vi "_23_Sample_qsns_10[3].vi"() -> ()   [LabVIEW 2020]
panel:
  out "s? t:f":dbl
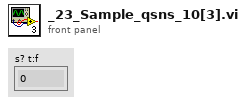
[diagram p1: front panel]
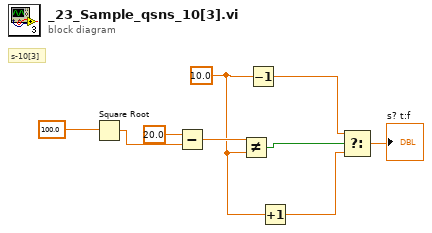
[diagram p0: block diagram]
diagram:
  w5 = 10.0 ("x")
  # "s-10[3]"
  n1 = Square Root(x=100.0) -> (sqrt(x)=w8:dbl)
  n2 = Subtract(x=20.0, y=w8) -> (x-y=w6:dbl)
  n3 = Not Equal?(x=w6, y=w5) -> (x != y?=w4:bool)
  n4 = Decrement(x=w5) -> (x-1=w3:dbl)
  n5 = Increment(x=w5) -> (x+1=w2:dbl)
  n6 = Select(t=w3, s=w4, f=w2) -> (s? t:f=→"s? t:f":dbl)
